vi "Show Package.vi"(7 "LabVIEW Web Service Request":refnum<class "Web Request.lvclass">, 10 "Name":string, 11 "Version":string) -> ()   [LabVIEW 2016]
uses:
  <vilib>/wsapi/Web Request.lvclass
  <vilib>/wsapi/class/subVIs/Write Single Session Variable.vi
  <vilib>/httpClient/LabVIEWHTTPClient.lvlib
panel:
  out "body":string
  out "headers":string
  out "resulting string":string
  # "Use the Web Service Request input terminal to call the VIs on the Web Services palette. Do not remove it from the connector pane unless you don't need access to the palette."
  # "Each additional control wired to the connector pane will be available as an input in the URL. To include an indicator in terminal-mode output (the default setting), it must also be wired to the connector pane."
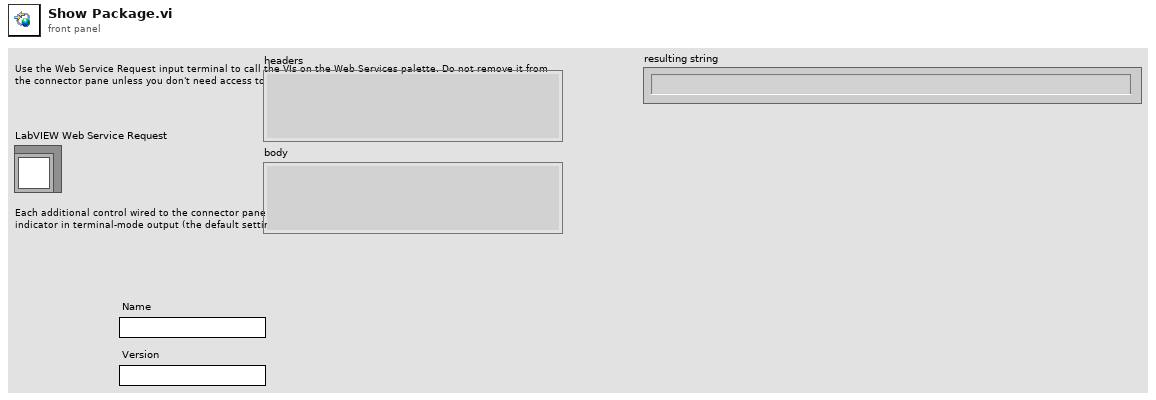
[diagram p1: front panel]
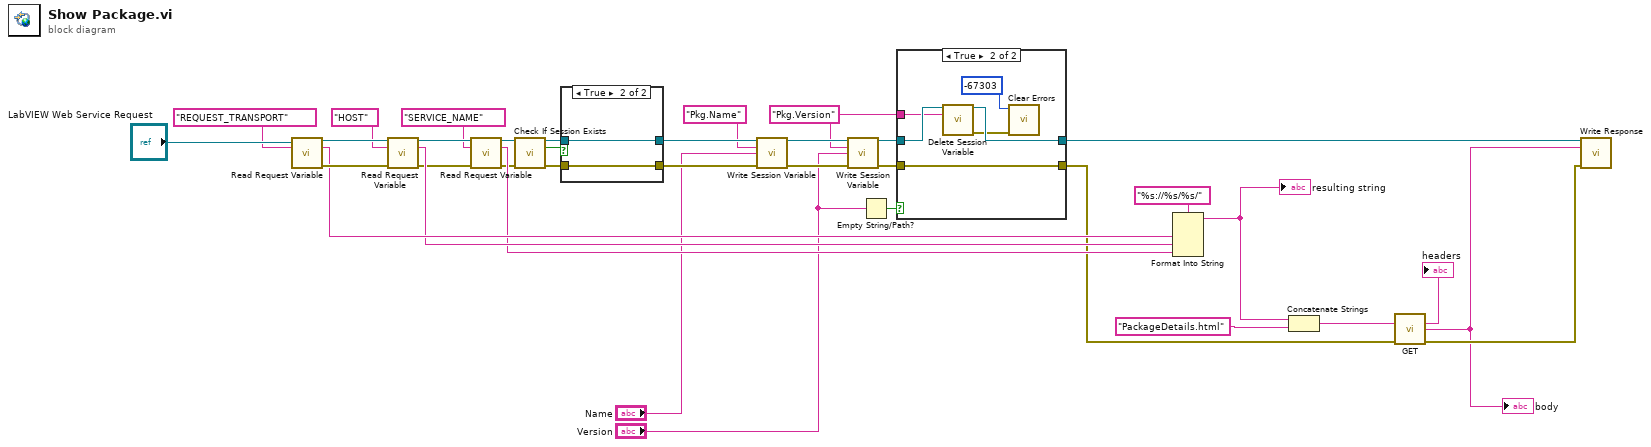
[diagram p0: block diagram]
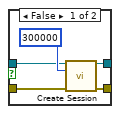
[diagram p3: hidden frame]
diagram:
  w1 = "Pkg.Version" ("key")
  n1 = call <vilib>:"Read Request Variable.vi"("LabVIEW Web Service Request"="LabVIEW Web Service Request", "variable name"="REQUEST_TRANSPORT") -> ("LabVIEW Web Service Request out"=w34:refnum<class "Web Request.lvclass">, "value"=w32:string, "error out"=w33:errorcluster)  [unwired: 11 in]
  n2 = call <vilib>:"Read Request Variable.vi"("LabVIEW Web Service Request"=w34, "variable name"="HOST", "error in (no error)"=w33) -> ("LabVIEW Web Service Request out"=w28:refnum<class "Web Request.lvclass">, "value"=w29:string, "error out"=w27:errorcluster)  [unwired: 10 in]
  n3 = call <vilib>:"Read Request Variable.vi"("LabVIEW Web Service Request"=w28, "variable name"="SERVICE_NAME", "error in (no error)"=w27) -> ("LabVIEW Web Service Request out"=w10:refnum<class "Web Request.lvclass">, "value"=w25:string, "error out"=w9:errorcluster)  [unwired: 10 in]
  n4 = call <vilib>:"Check If Session Exists.vi"("LabVIEW Web Service Request"=w10, "error in (no error)"=w9) -> ("LabVIEW Web Service Request out"=w12:refnum<class "Web Request.lvclass">, "session exists?"=w11:bool, "error out"=w13:errorcluster)  [unwired: 11 in]
  n5 = case shown="True" w11 {
    tunnel: [w40 w43] -> w18
    tunnel: [w39 w42] -> w17
    tunnel: w13 -> [w38 w42]
    tunnel: w12 -> [w37 w43]
    frame False {
      n6 = call <vilib>:"Create Session.vi"("LabVIEW Web Service Request"=w37, "timeout (60000 msec)"=u32 300000, "error in (no error)"=w38) -> ("LabVIEW Web Service Request out"=w40:refnum<class "Web Request.lvclass">, "error out"=w39:errorcluster)  [unwired: 10 in, 1 out]
    }
    frame True {
    }
  }
  n7 = call-poly <vilib>:"Write Session Variable.vi"("LabVIEW Web Service Request"=w18, "key"="Pkg.Name", "value"="Name", "error in (no error)"=w17) -> ("LabVIEW Web Service Request out"=w15:refnum<class "Web Request.lvclass">, "error out"=w14:errorcluster)  [unwired: 8 in, 2 out]
  n8 = call-poly <vilib>:"Write Session Variable.vi"("LabVIEW Web Service Request"=w15, "key"=w1, "value"="Version", "error in (no error)"=w14) -> ("LabVIEW Web Service Request out"=w7:refnum<class "Web Request.lvclass">, "error out"=w6:errorcluster)  [unwired: 8 in, 2 out]
  n9 = Empty String/Path?(string/path="Version") -> (empty?=w2:bool)
  n10 = case shown="True" w2 {
    tunnel: w6 -> [w44 w48]
    tunnel: [w44 w48] -> w4
    tunnel: w7 -> [w45 w51]
    tunnel: [w45 w50] -> w5
    tunnel: w1 -> [_ w49]
    frame False {
    }
    frame True {
      n11 = call <vilib>:"Delete Session Variable.vi"("LabVIEW Web Service Request"=w51, "key"=w49) -> ("LabVIEW Web Service Request out"=w50:refnum<class "Web Request.lvclass">, "error out"=w47:errorcluster)  [unwired: 12 in]
      n12 = call <vilib>:"Clear Errors.vi"("error in (no error)"=w47, "specific error code to clear (0: all)"=-67303) -> ()  [unwired: 4 in, 2 out]
    }
  }
  n13 = Format Into String(format string="%s://%s/%s/", w32, w29, w25) -> (resulting string=w19:string)  [unwired: 2 in, 1 out]
  "resulting string" <- w19
  n14 = Concatenate Strings(w19, "PackageDetails.html" ("string")) -> (w22:string)
  n15 = call <vilib>:"GET.vi"("url"=w22, "error in (no error)"=w4) -> ("headers"=→"headers":string, "body"=w20:string, "error out"=w24:errorcluster)  [unwired: 10 in, 1 out]
  "body" <- w20
  n16 = call <vilib>:"Write Response.vi"("LabVIEW Web Service Request"=w5, "response string"=w20, "error in (no error)"=w24) -> ()  [unwired: 11 in, 2 out]
